vi "Swerve Math.vi"(9 "Yaw":dbl, 10 "Rot. Point Y":dbl, 11 "Rot. Point X":dbl) -> (3 "Swerve Math Ouput":dbl[](array[numeric]))   [LabVIEW 2018]
uses:
  Drive Train Global.vi
  <vilib>/addons/control/pid/pid.llb/PID (DBL).vi
  Robot Information/Robot Information Global.vi
  <vilib>/addons/control/pid/NI_PID_pid.lvlib
panel:
  in  "Stop Rotation while translate":bool
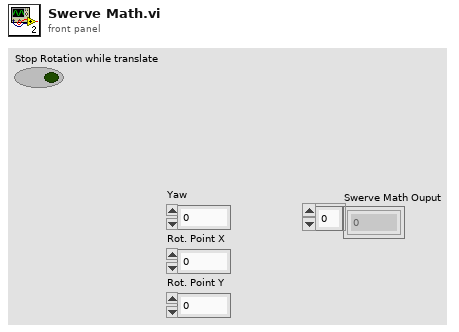
[diagram p1: front panel]
types:
  T1 = cluster{"Rollover":dbl, "Yaw":dbl, "Cont Yaw":dbl}
  T2 = cluster{"proportional gain (Kc)":dbl, "integral time (Ti, min)":dbl, "derivative time (Td, min)":dbl}
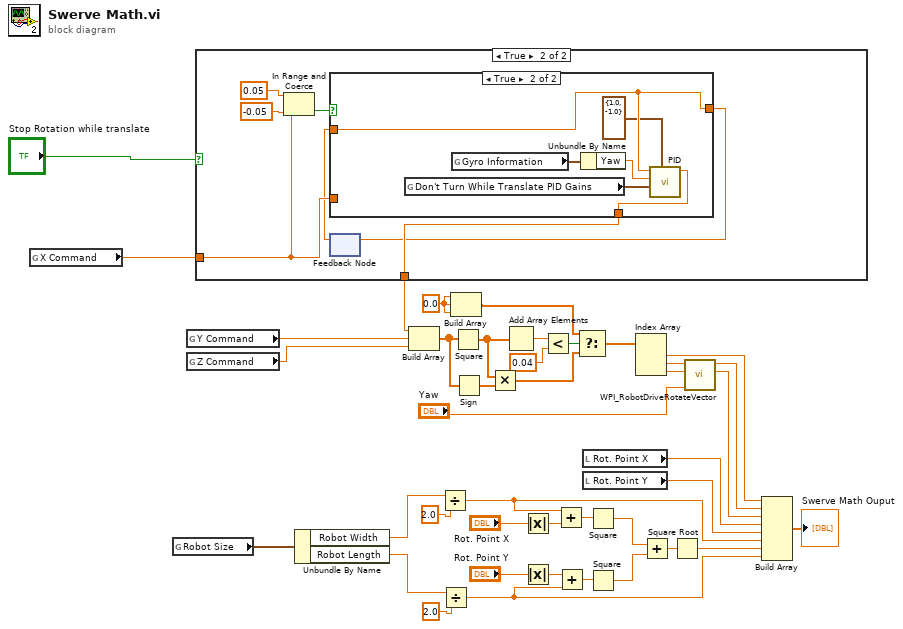
[diagram p0: block diagram]
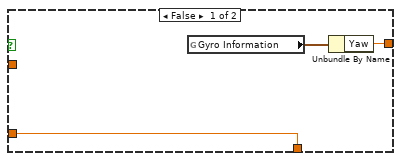
[diagram p3: hidden frame]
diagram:
  w11 = 0.0 ("element")
  n1 = global read "Drive Train Global.vi" "X Command"() -> (w2:dbl)
  n2 = global read "Robot Information Global.vi" "Robot Size"() -> (w18:cluster{"Robot Width":dbl, "Robot Length":dbl})
  n3 = global read "Drive Train Global.vi" "Y Command"() -> (w5:dbl)
  n4 = global read "Drive Train Global.vi" "Z Command"() -> (w19:dbl)
  n5 = case shown="True" "Stop Rotation while translate" {
    tunnel: [w42 w46] -> w3
    tunnel: w2 -> [w42 w45]
    frame False {
    }
    frame True {
      n6 = In Range and Coerce(upper limit=0.05, x=w45, lower limit=-0.05) -> (In Range?=w49:bool)  [unwired: 1 out]
      n7 = feedback #1() -> (w44:dbl)  [unwired: 1 in]
      n8 = case shown="True" w49 {
        tunnel: [w52 w53] -> w46
        tunnel: w45 -> [w52 _]
        tunnel: w44 -> [_ w58]
        tunnel: [w50 w58] -> w43
        frame False {
          n9 = global read "Drive Train Global.vi" "Gyro Information"() -> (w51:T1)
          n10 = Unbundle By Name(w51) -> ("Yaw"=w50:dbl)
        }
        frame True {
          n11 = global read "Drive Train Global.vi" "Don't Turn While Translate PID Gains"() -> (w54:T2)
          n12 = global read "Drive Train Global.vi" "Gyro Information"() -> (w57:T1)
          n13 = Unbundle By Name(w57) -> ("Yaw"=w56:dbl)
          n14 = call-poly <vilib>:"PID.vi"("output range"=cluster{"output high":dbl, "output low":dbl} {"output high"=1.0, "output low"=-1.0}, "PID gains"=w54, "process variable"=w56, "setpoint"=w58) -> ("output"=w53:dbl)  [unwired: 6 in, 1 out]
        }
      }
      n15 = feedback-in #1(w43) -> ()
    }
  }
  n16 = Unbundle By Name(w18) -> ("Robot Width"=w16:dbl, "Robot Length"=w17:dbl)
  n17 = Build Array(w3, w5, w19) -> (w7:dbl[])
  n18 = Divide(x=w16, y=2.0) -> (x/y=w27:dbl)
  n19 = Divide(x=w17, y=2.0) -> (x/y=w25:dbl)
  n20 = Build Array(w11, w11, w11) -> (w12:dbl[])
  n21 = Square(x=w7) -> (x^2=w9:dbl[])
  n22 = Sign(1:w7) -> (0:w10:dbl[])
  n23 = Multiply(x=w9, y=w10) -> (x*y=w8:dbl[])
  n24 = Add Array Elements(numeric array=w9) -> (sum=w15:dbl)
  n25 = Absolute Value(x="Rot. Point X") -> (abs(x)=w41:dbl)
  n26 = Absolute Value(x="Rot. Point Y") -> (abs(x)=w39:dbl)
  n27 = Less?(x=w15, y=0.04 ("x")) -> (x < y?=w13:bool)
  n28 = Add(x=w27, y=w41) -> (x+y=w40:dbl)
  n29 = Add(x=w39, y=w25) -> (x+y=w38:dbl)
  n30 = Select(t=w12, s=w13, f=w8) -> (s? t:f=w23:dbl[])
  n31 = local read "Rot. Point X"() -> (w29:dbl)
  n32 = local read "Rot. Point Y"() -> (w28:dbl)
  n33 = Square(x=w40) -> (x^2=w36:dbl)
  n34 = Square(x=w38) -> (x^2=w37:dbl)
  n35 = Index Array(array=w23) -> (element #1=w21:dbl, element #2=w24:dbl, element #3=w30:dbl)  [unwired: 3 in]
  n36 = Add(x=w36, y=w37) -> (x+y=w35:dbl)
  n37 = Square Root(x=w35) -> (sqrt(x)=w26:dbl)
  n38 = call <vilib>:"WPI_RobotDriveRotateVector.vi"("Angle"="Yaw", "X"=w30, "Y"=w24) -> ("X'"=w22:dbl, "Y'"=w20:dbl)  [unwired: 7 out]
  n39 = Build Array(w21, w20, w22, w29, w28, w27, w26, w25) -> (→"Swerve Math Ouput":dbl[])
